vi "Get Devices In Family.vi"(8 "Error In":errorcluster, 11 "Family Index":i32) -> (0 "Error Out":errorcluster, 3 "Devices":string[](array[string]))   [LabVIEW 2020, in "LMH-LINX.lvlib"]
uses:
  LMH-LINX.lvlib
  Type Defs/All Firmware Data FGV States.ctl
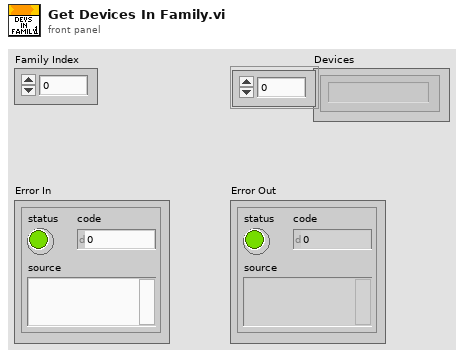
[diagram p1: front panel]
types:
  T1 = typedef "LMH-LINX.lvlib/All Firmware Data FGV States.ctl" = enum16{"Set", "Get"}
  T2 = typedef "LMH-LINX.lvlib/Device Data.ctl" = cluster{"Family ID":i32, "Family Name":string, "Device ID":i32, "Device Name":string, "Firmware Program Interfaces":string[], "Path":path}
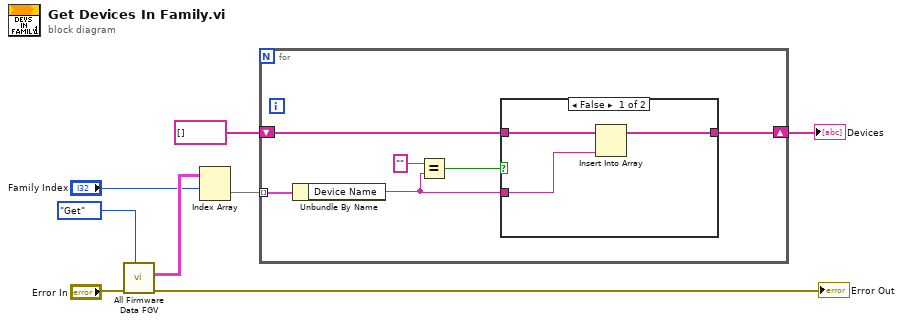
[diagram p0: block diagram]
diagram:
  n1 = call "All Firmware Data FGV.vi"("All Firmware Data FGV States"=All_Firmware_Data_FGV_States."Get", "Error In"="Error In") -> ("Error Out"=→"Error Out":errorcluster, "Devices"=w7:T2[][])  [unwired: 6 in, 2 out]
  n2 = Index Array(array=w7, index (row)="Family Index") -> (element=w3:T2[])  [unwired: 1 in]
  n3 = for {
    tunnel: w3 -> [w14] mode=indexing
    shift-right: [w10] -> w1
    shift-left: string[] [] ("Devices") -> [w11]
    n4 = Unbundle By Name(w14) -> ("Device Name"=w9:string)
    n5 = Equal?(x="", y=w9) -> (x = y?=w12:bool)
    n6 = case shown="False" w12 {
      tunnel: w11 -> [w17 w18]
      tunnel: [w16 w18] -> w10
      tunnel: w9 -> [w15 _]
      frame False {
        n7 = Insert Into Array(array=w17, new element=w15) -> (w16:string[])  [unwired: 1 in]
      }
      frame True {
      }
    }
  }
  "Devices" <- w1
